vi "MT Set Axis Halt.vi"(11 "AObj":u16) -> (3 "function return":i32)   [LabVIEW 2014, in "MT_API.lvlib"]
doc: "MT_API INT32 __stdcall MT_Set_Axis_Halt(WORD AObj);"
uses:
  MT_API.lvlib
  MT_API.dll
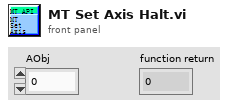
[diagram p1: front panel]
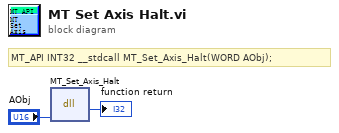
[diagram p0: block diagram]
diagram:
  # "MT_API INT32 __stdcall MT_Set_Axis_Halt(WORD AObj);"
  n1 = dll-call lib="E:/Projects/LabView/MT_API/MT_API.*" fn="MT_Set_Axis_Halt"("AObj"="AObj") -> (→"function return":i32)  [unwired: 4 in, 2 out]
